vi "Read Log_odd_sensor_parameters.vi"(8 "error in (no error)":errorcluster, 11 "Probabilistic_OccupancyGrid in":refnum<class "Probabilistic_OccupancyGrid.lvclass">) -> (0 "error out":errorcluster, 1 "Log_odd_sensor_negative_detection":dbl, 2 "Log_odd_sensor_positive_detection":dbl, 3 "Probabilistic_OccupancyGrid out":refnum<class "Probabilistic_OccupancyGrid.lvclass">)   [LabVIEW 2017, in "Probabilistic_OccupancyGrid.lvclass"]
uses:
  Probabilistic_OccupancyGrid.lvclass
  Probabilistic_OccupancyGrid.lvclass/Probabilistic_OccupancyGrid.ctl
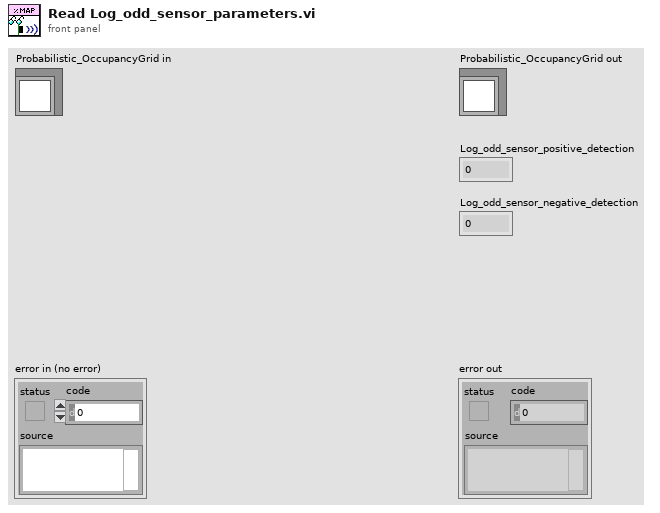
[diagram p1: front panel]
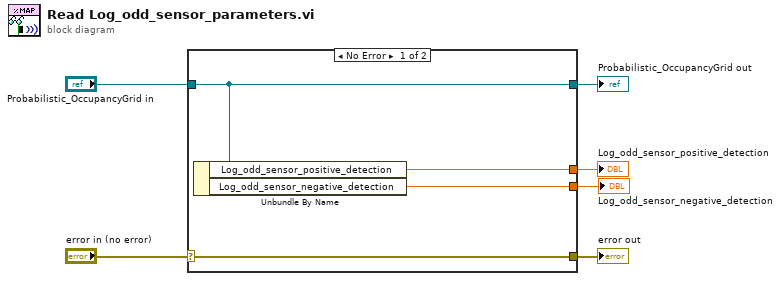
[diagram p0: block diagram]
diagram:
  n1 = case shown="No Error" "error in (no error)" {
    selector: "error in (no error)" -> [w10 w11]
    tunnel: [w10 w11] -> w5
    tunnel: [w9 w12] -> w3
    tunnel: "Probabilistic_OccupancyGrid in" -> [w9 w12]
    tunnel: [w8 _] -> w2
    tunnel: [w7 _] -> w1
    frame No Error {
      n2 = Unbundle By Name(w9) -> ("Log_odd_sensor_positive_detection"=w8:dbl, "Log_odd_sensor_negative_detection"=w7:dbl)
    }
    frame Error {
    }
  }
  "error out" <- w5
  "Probabilistic_OccupancyGrid out" <- w3
  "Log_odd_sensor_positive_detection" <- w2
  "Log_odd_sensor_negative_detection" <- w1
